vi "bitrate e2n.vi"(1 "enum":T1=enum."RATE_1Mbps") -> (0 "number":u16 format="%0d")   [LabVIEW 2024, in "atsj peakcan basic.lvlib"]
uses:
  bitrate.ctl
  atsj peakcan basic.lvlib
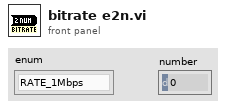
[diagram p1: front panel]
types:
  T1 = typedef "atsj peakcan basic.lvlib/bitrate.ctl" = enum16{"RATE_UNSUPPORTED", "RATE_1Mbps", "RATE_800kbps", "RATE_500kbps", "RATE_250kbps", "RATE_125kbps", "RATE_100kbps", "RATE_95kbps", "RATE_83kbps", "RATE_50kbps", "RATE_47kbps", "RATE_33kbps", "RATE_20kbps", "RATE_10kbps", "RATE_5kbps"}
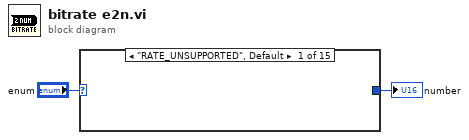
[diagram p0: block diagram]
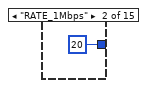
[diagram p2: hidden frame]
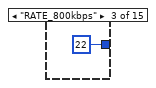
[diagram p3: hidden frame]
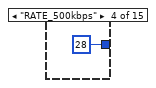
[diagram p4: hidden frame]
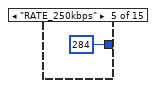
[diagram p5: hidden frame]
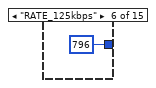
[diagram p6: hidden frame]
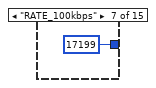
[diagram p7: hidden frame]
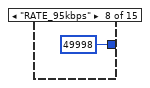
[diagram p8: hidden frame]
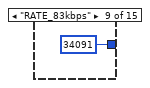
[diagram p9: hidden frame]
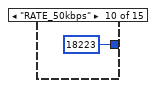
[diagram p10: hidden frame]
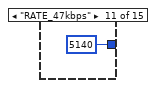
[diagram p11: hidden frame]
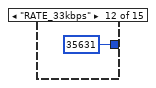
[diagram p12: hidden frame]
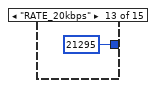
[diagram p13: hidden frame]
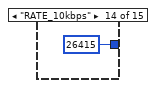
[diagram p14: hidden frame]
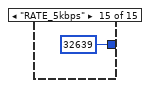
[diagram p15: hidden frame]
diagram:
  n1 = case shown="\"RATE_UNSUPPORTED\", Default" "enum" {
    tunnel: [_ u16 20 u16 22 u16 28 u16 284 u16 796 u16 17199 u16 49998 u16 34091 u16 18223 u16 5140 u16 35631 u16 21295 u16 26415 u16 32639] -> w1
    frame "RATE_UNSUPPORTED", Default {
    }
    frame "RATE_1Mbps" {
    }
    frame "RATE_800kbps" {
    }
    frame "RATE_500kbps" {
    }
    frame "RATE_250kbps" {
    }
    frame "RATE_125kbps" {
    }
    frame "RATE_100kbps" {
    }
    frame "RATE_95kbps" {
    }
    frame "RATE_83kbps" {
    }
    frame "RATE_50kbps" {
    }
    frame "RATE_47kbps" {
    }
    frame "RATE_33kbps" {
    }
    frame "RATE_20kbps" {
    }
    frame "RATE_10kbps" {
    }
    frame "RATE_5kbps" {
    }
  }
  "number" <- w1
